vi "Active Outtake Loop.vi"   [LabVIEW 2016]
uses:
  Common Code/Utilities/Change Detect Boolean.vi
  Robot Global Data.vi
  <vilib>/Rock Robotics/WPI/Solenoid/Deprecated/WPI_SolenoidSetBool.vi
types:
  T1 = typedef "Intake Control Cluster.ctl" = cluster{"Intake Mode":T2, "Intake Auto Command":T3, "Intake Current Trip State":T4, "Flap Open? / Confirm Outtake?":bool, "Engage traction for gear load?":bool, "Wings open?":bool, "Manual Intake Power":dbl, "Outtake?":bool, "Unload State":T5, "Load State":T6, "Unload Mode":T7}
  T2 = typedef "Intake Modes.ctl" = enum16{"Manual", "Auto"}
  T3 = typedef "Intake Auto States.ctl" = enum16{"Outtake", "Idle", "Intake", "Intake Pull Up"}
  T4 = typedef "Intake Trip States.ctl" = enum16{"Normal", "Backward Tripped", "Forward Tripped"}
  T5 = typedef "Outtake State.ctl" = enum16{"Idle", "Start", "Doors Open", "Push Out"}
  T6 = typedef "Load State.ctl" = enum16{"Idle", "Open Flap", "Ready Close", "Ready Far"}
  T7 = typedef "Unload Mode.ctl" = enum16{"None", "Close", "Far"}
  T8 = typedef "Dashboard Control Data.ctl" = cluster{"Drivetrain Settings":T9, "Intake Presets ":T12, "Shooter Presets":T13, "Vision Target Packet":T14, "Auton Presets":cluster{"Start Position":dbl}, "Drivetrain Encoder Values":T15, "Drivetrain Encoder Settings":cluster{"Left Tick Constant":dbl, "Right Tick Contant":dbl, "Reset Encoders":bool, "Center Tick Constant":dbl}, "Zero Gyro":bool, "Vision Timeout":dbl, "Pressure M":dbl, "Pressure B":dbl, "Auto Agitator":T17, "Climber Settings":T18, "LEDs":T19}
  T9 = typedef "Drivetrain Settings.ctl" = cluster{"Gyro Tolerance":dbl, "Gyro Steer PID Gains":T10, "Y Power Multiplier":dbl, "Turn Power Multiplier":dbl, "Gyro Output":dbl, "Creep Rate":dbl, "Distance Drive PID Gains":T10, "Distance Tolerance":dbl, "Distance Output":dbl, "Strafe Threshold":dbl, "Strafe Correct":bool, "Strafe Tolerance":dbl, "Translate Drive PID Gains":T10, "Strafe Output":dbl, "SC Right":dbl, "SC Left":dbl, "Use Gyro":bool, "Constant Power":bool, "Strafe Power":dbl, "Input Modifier":T11, "SCR Delay":dbl, "SCL Delay":dbl}
  T10 = typedef "PID Gains.ctl" = cluster{"proportional gain (Kc)":dbl, "integral time (Ti, min)":dbl, "derivative time (Td, min)":dbl}
  T11 = typedef "Input Modifier.ctl" = enum16{"None", "Square", "Cube"}
  T12 = typedef "Intake Presets.ctl" = cluster{"Intake Speed ":dbl, "Outake Speed":dbl, "Current Trip Delay":dbl, "Max Current":dbl, "Gear Outtake Motor Delay":dbl, "Gear Intake Motor Delay":dbl, "Gear Intake?":bool, "Gear Intake Pull Up Speed":dbl, "Pusher Delay":dbl, "Release Delay":dbl, "Close Release Delay":dbl}
  T13 = typedef "Shooter Presets.ctl" = cluster{"Key Shot":cluster{"RPM ":dbl, "Hood?":bool}, "Distance Shot":cluster{"RPM":dbl, "Hood?":bool}, "RPM Tolerance":dbl, "Unstuck Delay Time ":dbl, "Initial RPM Increase":dbl, "Warmup Delay":dbl, "Faster Time":dbl, "Shooter PID Gains":cluster{"P":dbl, "I":dbl, "D":dbl, "FF":dbl, "Ramp Rate":dbl, "I Zone":dbl}, "Unstuck Trigger Power":dbl, "Trigger Power":dbl, "Unstuck RPM":dbl, "Agitator Active Power":dbl, "Agitator Idle Power":dbl, "RPM Tuning Range":dbl, "RPM M Tuning Range":dbl}
  T14 = typedef "Vision Target Packet.ctl" = cluster{"Robot Center":dbl, "Center X":dbl, "Center Y":dbl, "Angle":dbl, "Distance":dbl, "Found Target?":bool}
  T15 = typedef "Drivetrain Encoder Values.ctl" = cluster{"Left Encoder":T16, "Center Encoder":T16, "Right Encoder":T16}
  T16 = typedef "Encoder Values.ctl" = cluster{"Distance":dbl, "Speed":dbl, "Tick":dbl}
  T17 = typedef "Auto Agitator Settings.ctl" = cluster{"Enable Auto Agitation":bool, "Continuous Stir":bool, "Continuous Intake":bool, "Alternate In/Outtake":bool, "Wing Delay":dbl, "Stir Delay":dbl, "Intake Delay":dbl, "Wing On Time":dbl, "Wing Off Time":dbl, "Stir On Time":dbl, "Stir Off Time":dbl, "Intake On Time":dbl, "Intake Off Time":dbl, "Stir Power":dbl, "Intake Power":dbl, "Outtake Power":dbl, "Intake Run Time":dbl, "Outtake Run Time":dbl, "Wing$":bool, "Intake":bool, "Stirrer":bool}
  T18 = typedef "Climber Settings.ctl" = cluster{"Climber Power":dbl, "Max Current":dbl, "Avoid Current Trip?":bool}
  T19 = typedef "LED Global Data.ctl" = cluster{"Back":cluster{"Default":string, "Traction":string, "Gear Ready":string, "Break On":string, "Gear Loaded":string, "Climb":string}, "Front":cluster{"Default":string, "Traction":string, "Gear Ready":string, "Break On":string, "Gear Loaded":string, "Climb":string}, "LEDOnTime":dbl, "LEDOffTime":dbl}
  T20 = typedef "Intake Status Cluster.ctl" = cluster{"Roller Power":dbl, "Intake Mode":T2, "Intake Auto State":T3, "Backward Tripped?":bool, "Forward Tripped?":bool, "Intake Current Trip State":T4, "Gear Flap Open":bool, "Doors Open":bool, "Traction for Gear?":bool, "Current Over Max Current?":bool, "Tripped?":bool, "Current":dbl, "Intake Down?":bool, "Gear Loaded":bool, "Pusher Activated":bool, "Outtake State":T5, "Load State":T6, "Unload Mode":T7}
  T21 = typedef "WPI_SolenoidDevRef.ctl" = cluster{"DevStatus":errorcluster, "Pneumatics Control Module":u8, "Forward Solenoid Channel":T22, "Reverse Solenoid Channel":T22}
  T22 = typedef "WPI_SolenoidChannel.ctl" = enum8{"Solenoid 0", "Solenoid 1", "Solenoid 2", "Solenoid 3", "Solenoid 4", "Solenoid 5", "Solenoid 6", "Solenoid 7", "Invalid"}
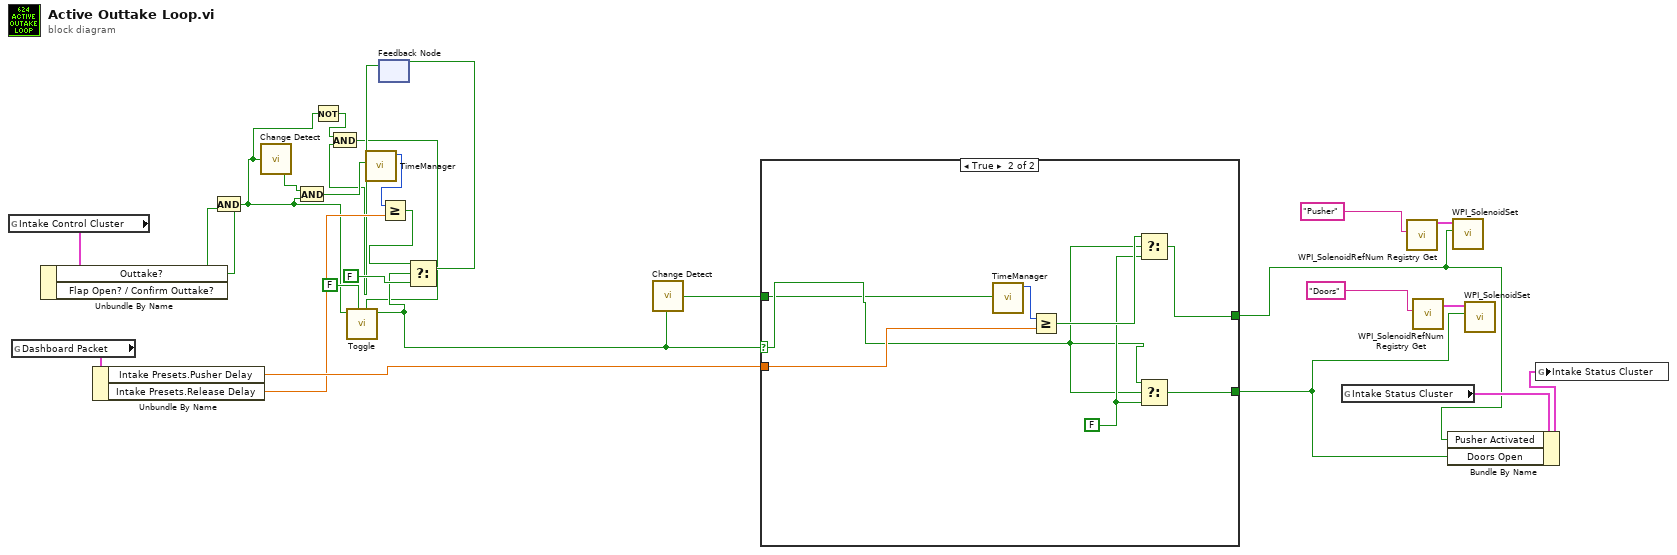
[diagram p0: block diagram]
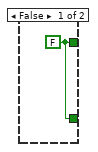
[diagram p2: hidden frame]
diagram:
  n1 = global read "Robot Global Data.vi" "Intake Control Cluster"() -> (w25:T1)
  n2 = global read "Robot Global Data.vi" "Dashboard Packet"() -> (w20:T8)
  n3 = Unbundle By Name(w25) -> ("Outtake?"=w24:bool, "Flap Open? / Confirm Outtake?"=w23:bool)
  n4 = Unbundle By Name(w20) -> ("Intake Presets.Pusher Delay"=w19:dbl, "Intake Presets.Release Delay"=w14:dbl)
  n5 = And(x=w24, y=w23) -> (x .and. y?=w4:bool)
  n6 = call-poly "Change Detect.vi"("In"=w4) -> ("Changed?"=w13:bool)
  n7 = And(x=w13, y=w4) -> (x .and. y?=w12:bool)
  n8 = Not(x=w4) -> (.not. x?=w3:bool)
  n9 = call "TimeManager.vi"("Reset?"=w12) -> ("Time Since Reset"=w11:u32)  [unwired: 9 in, 1 out]
  n10 = feedback #1() -> (w2:bool)  [unwired: 1 in]
  n11 = And(x=w3, y=w2) -> (x .and. y?=w1:bool)
  n12 = call "Toggle.vi"("Reinit?"=w1, "Initial Value"=FALSE, "In"=w4) -> ("Toggled"=w6:bool)  [unwired: 8 in]
  n13 = Greater Or Equal?(x=w11, y=w14) -> (x >= y?=w9:bool)
  n14 = Select(t=w9, s=w6, f=FALSE) -> (s? t:f=w8:bool)
  n15 = feedback-in #1(w8) -> ()
  n16 = call-poly "Change Detect.vi"("In"=w6) -> ("Changed?"=w5:bool)
  n17 = case shown="True" w6 {
    selector: w6 -> [_ w30]
    tunnel: w19 -> [_ w36]
    tunnel: [w28 w33] -> w16
    tunnel: [w28 w32] -> w15
    tunnel: w5 -> [_ w29]
    frame False {
      w28 = FALSE
    }
    frame True {
      w31 = FALSE
      n18 = call "TimeManager.vi"("Reset?"=w29) -> ("Time Since Reset"=w35:u32)  [unwired: 9 in, 1 out]
      n19 = Greater Or Equal?(x=w35, y=w36) -> (x >= y?=w34:bool)
      n20 = Select(t=w34, s=w30, f=w31) -> (s? t:f=w33:bool)
      n21 = Select(t=w30, s=w30, f=w31) -> (s? t:f=w32:bool)
    }
  }
  n22 = global read "Robot Global Data.vi" "Intake Status Cluster"() -> (w18:T20)
  n23 = call <vilib>:"WPI_SolenoidRefNum Registry Get.vi"("refnum name"="Pusher") -> ("SolenoidDevRef"=w27:T21)  [unwired: 9 in, 1 out]
  n24 = call <vilib>:"WPI_SolenoidRefNum Registry Get.vi"("refnum name"="Doors") -> ("SolenoidDevRef"=w21:T21)  [unwired: 9 in, 1 out]
  n25 = Bundle By Name(cluster=w18, "Pusher Activated"=w16, "Doors Open"=w15) -> (w17:T20)
  n26 = call-poly <vilib>:"WPI_SolenoidSet.vi"("Value"=w16, "SolenoidDevRef"=w27) -> ()  [unwired: 8 in, 2 out]
  n27 = call-poly <vilib>:"WPI_SolenoidSet.vi"("Value"=w15, "SolenoidDevRef"=w21) -> ()  [unwired: 8 in, 2 out]
  n28 = global write "Robot Global Data.vi" "Intake Status Cluster"(w17) -> ()
